vi "Create Rendezvous.vi"(4 "error in (no error)":errorcluster, 5 "return existing (F)":bool, 6 "size (2)":i32=2, 7 "name (unnamed)":string) -> (0 "error out":errorcluster, 1 "created new":bool, 3 "rendezvous":T1)   [LabVIEW 2010]
doc: "Looks up an existing rendezvous or creates a new rendezvous and returns a refnum."
uses:
  Rendezvous Name & Ref DB Action.ctl
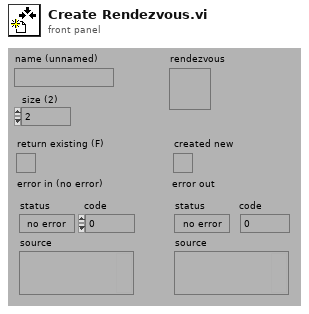
[diagram p1: front panel]
types:
  T1 = typedef "Rendezvous RefNum" = refnum<k1>
  T2 = typedef "Rendezvous Name & Ref DB Action.ctl" = enum16{"Lookup", "Insert", "Remove"}
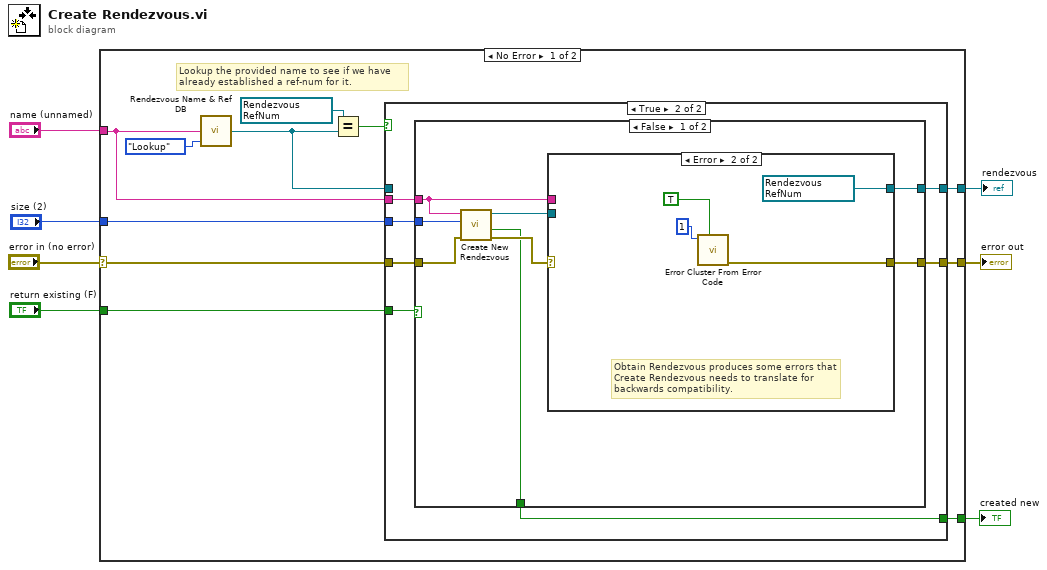
[diagram p0: block diagram]
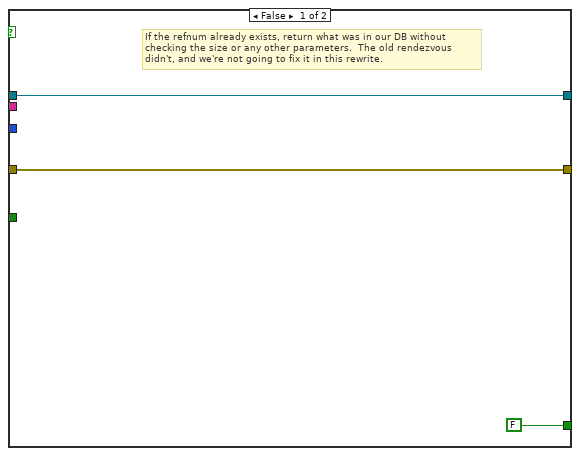
[diagram p2: hidden frame]
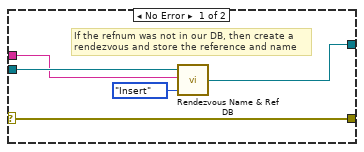
[diagram p3: hidden frame]
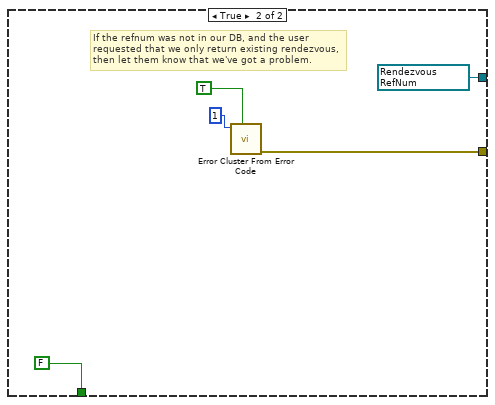
[diagram p4: hidden frame]
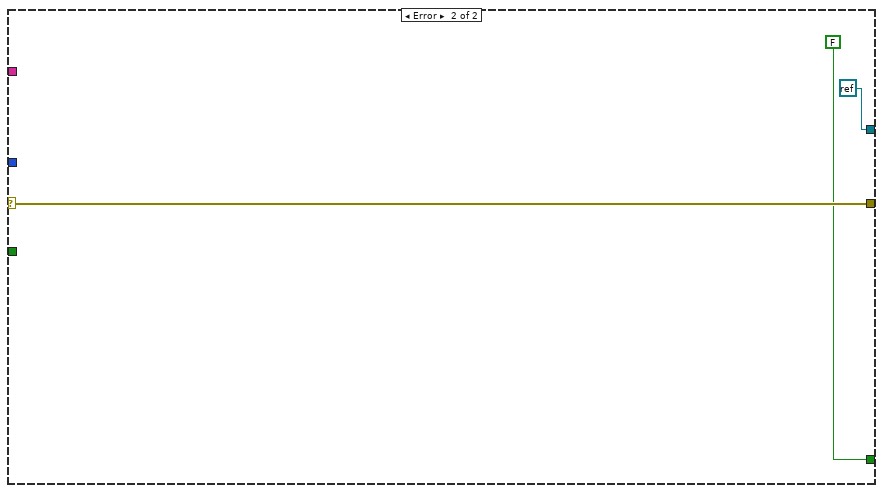
[diagram p5: hidden frame]
diagram:
  n1 = case shown="No Error" "error in (no error)" {
    selector: "error in (no error)" -> [w13 w53]
    tunnel: "name (unnamed)" -> [w9 _]
    tunnel: "size (2)" -> [w16 _]
    tunnel: "return existing (F)" -> [w17 _]
    tunnel: [w18 FALSE] -> w5
    tunnel: [w14 w53] -> w3
    tunnel: [w12 refnum<k0> refnum] -> w2
    frame No Error {
      w8 = T1 refnum items=["rendezvous"] ("x")
      # "Lookup the provided name to see if we have already established a ref-num for it."
      n2 = call "Rendezvous Name & Ref DB.vi"("Action"=Rendezvous_Name_&_Ref_DB_Action."Lookup" ("Semaphore Name & Ref DB Action"), "Rendezvous Name"=w9) -> ("rendezvous  ref out"=w10:T1)  [unwired: 1 in]
      n3 = Equal?(x=w8, y=w10) -> (x = y?=w15:bool)
      n4 = case shown="True" w15 {
        tunnel: w9 -> [_ w24]
        tunnel: [FALSE ("created new") w27] -> w18
        tunnel: w17 -> [_ w22]
        tunnel: w16 -> [_ w25]
        tunnel: [w21 w28] -> w14
        tunnel: w13 -> [w21 w26]
        tunnel: w10 -> [w19 _]
        tunnel: [w19 w23] -> w12
        frame False {
          # "If the refnum already exists, return what was in our DB without checking the size or any other parameters.  The old rendezvous didn't, and we're not going to fix it in this rewrite."
        }
        frame True {
          n5 = case shown="False" w22 {
            tunnel: [w36 w48] -> w28
            tunnel: [w34 FALSE] -> w27
            tunnel: w26 -> [w33 _]
            tunnel: w25 -> [w32 _]
            tunnel: w24 -> [w29 _]
            tunnel: [w31 w46] -> w23
            frame False {
              n6 = call "Create New Rendezvous.vi"("error in (no error)"=w33, "size (2)"=w32, "name (unnamed)"=w29) -> ("error out"=w35:errorcluster, "created new"=w34:bool, "rendezvous"=w30:T1)  [unwired: 1 in, 1 out]
              n7 = case shown="Error" w35 {
                selector: w35 -> [w41 _]
                tunnel: [w41 w45] -> w36
                tunnel: [w37 w42] -> w31
                tunnel: w30 -> [w39 _]
                tunnel: w29 -> [w38 _]
                frame No Error {
                  # "If the refnum was not in our DB, then create a rendezvous and store the reference and name"
                  n8 = call "Rendezvous Name & Ref DB.vi"("Action"=Rendezvous_Name_&_Ref_DB_Action."Insert" ("Semaphore Name & Ref DB Action"), "Rendezvous Name"=w38, "rendezvous ref in"=w39) -> ("rendezvous  ref out"=w37:T1)
                }
                frame Error {
                  w42 = T1 refnum items=["rendezvous"] ("rendezvous  ref out")
                  # "Obtain Rendezvous produces some errors that Create Rendezvous needs to translate for backwards compatibility."
                  n9 = call "Error Cluster From Error Code.vi"("show call chain? (False)"=TRUE, "error code (0)"=1) -> ("error out"=w45:errorcluster)  [unwired: 1 in, 6 out]
                }
              }
            }
            frame True {
              w46 = T1 refnum items=["rendezvous"] ("rendezvous  ref out")
              # "If the refnum was not in our DB, and the user requested that we only return existing rendezvous, then let them know that we've got a problem."
              n10 = call "Error Cluster From Error Code.vi"("show call chain? (False)"=TRUE, "error code (0)"=1) -> ("error out"=w48:errorcluster)  [unwired: 1 in, 6 out]
            }
          }
        }
      }
    }
    frame Error {
    }
  }
  "error out" <- w3
  "rendezvous" <- w2
  "created new" <- w5
